vi "Revision Query.vi"(8 "error in (no error)":errorcluster, 11 "VISA resource name":refnum<visa-resource-name>) -> (0 "error out":errorcluster, 1 "Instrument Firmware Revision":string, 2 "Instrument Driver Revision":string, 3 "VISA resource name out":refnum<visa-resource-name>)   [LabVIEW 2018, in "Keithley 3706.lvlib"]
uses:
  <instrlib>/Keithley 3706/Keithley 3706.lvlib
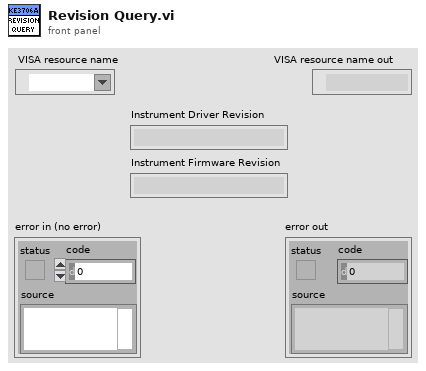
[diagram p1: front panel]
types:
  T1 = enum32{"invalid app kind", "Development System", "Run Time System", "Student Edition", "Embedded LabVIEW", "Evaluation", "Custom"}
  T2 = cluster{"Major":u16, "Minor":u16, "Fix":u16, "Build":u16}
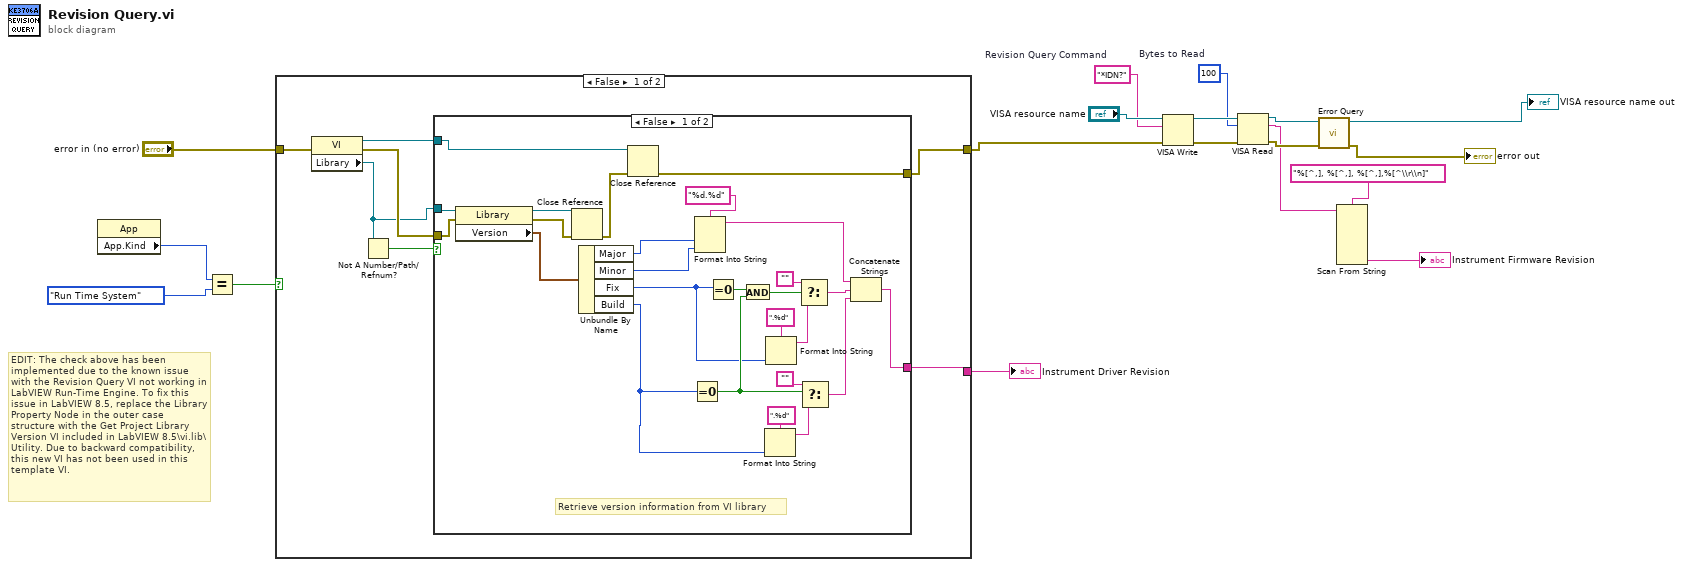
[diagram p0: block diagram]
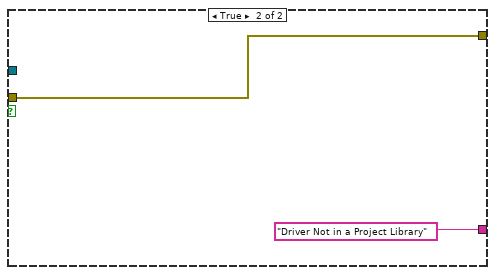
[diagram p2: hidden frame]
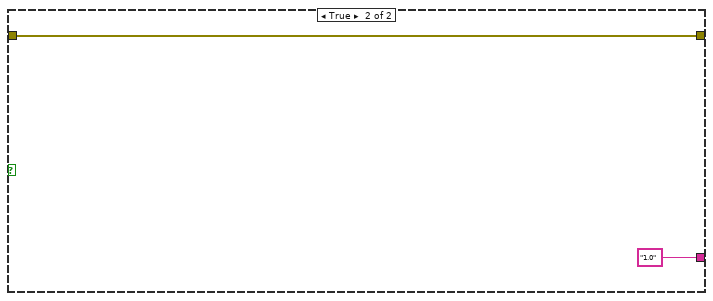
[diagram p3: hidden frame]
diagram:
  w8 = u32 100  # Bytes to Read
  w11 = "*IDN?"  # Revision Query Command
  # "EDIT: The check above has been implemented due to the known issue with the Revision Query VI not working in LabVIEW Run-Time Engine. To fix this issue in LabVIEW 8.5, replace the Library Property Node in the outer case structure with the Get Project Library Version VI included in LabVIEW 8.5\\vi.lib\\Utility. Due to backward compatibility, this new VI has not been used in this template VI."
  n1 = property class="App"() -> ("App.Kind"=w18:T1)  [unwired: 2 in, 2 out]
  n2 = Equal?(x=w18, y=T1."Run Time System" ("Application:Kind")) -> (x = y?=w16:bool)
  n3 = case shown="False" w16 {
    tunnel: "error in (no error)" -> [w25 w55]
    tunnel: [w20 w55] -> w13
    tunnel: [w21 "1.0"] -> w14
    frame False {
      n4 = property class="VI"(error in=w25) -> (reference out=w24:refnum<vi>, error out=w23:errorcluster, "Library"=w19:refnum<vi>)  [unwired: 1 in]
      n5 = Not A Number/Path/Refnum?(number/path/refnum=w19) -> (NaN/Path/Refnum?=w22:bool)
      n6 = case shown="False" w22 {
        tunnel: w24 -> [w47 _]
        tunnel: w23 -> [w51 w53]
        tunnel: [w45 w53] -> w20
        tunnel: [w39 "Driver Not in a Project Library"] -> w21
        tunnel: w19 -> [w50 _]
        frame False {
          # "Retrieve version information from VI library"
          n7 = property class="Library"(reference=w50, error in=w51) -> (reference out=w49:refnum<vi>, error out=w48:errorcluster, "Version"=w43:T2)
          n8 = Close Reference(reference=w49, error in (no error)=w48) -> (error out=w46:errorcluster)
          n9 = Unbundle By Name(w43) -> ("Major"=w42:u16, "Minor"=w41:u16, "Fix"=w28:u16, "Build"=w29:u16)
          n10 = Close Reference(reference=w47, error in (no error)=w46) -> (error out=w45:errorcluster)
          n11 = Equal To 0?(x=w29) -> (x = 0?=w37:bool)
          n12 = Format Into String(format string="%d.%d", w42, w41) -> (resulting string=w40:string)  [unwired: 2 in, 1 out]
          n13 = Equal To 0?(x=w28) -> (x = 0?=w36:bool)
          n14 = And(x=w36, y=w37) -> (x .and. y?=w38:bool)
          n15 = Format Into String(format string=".%d", w29) -> (resulting string=w33:string)  [unwired: 2 in, 1 out]
          n16 = Format Into String(format string=".%d", w28) -> (resulting string=w32:string)  [unwired: 2 in, 1 out]
          n17 = Select(t="", s=w38, f=w32) -> (s? t:f=w27:string)
          n18 = Select(t="", s=w37, f=w33) -> (s? t:f=w26:string)
          n19 = Concatenate Strings(w40, w27, w26) -> (w39:string)
        }
        frame True {
        }
      }
    }
    frame True {
    }
  }
  "Instrument Driver Revision" <- w14
  n20 = VISA Write(VISA resource name="VISA resource name", write buffer=w11, error in (no error)=w13) -> (VISA resource name out=w9:refnum<visa-resource-name>, error out=w10:errorcluster)  [unwired: 1 out]
  n21 = VISA Read(VISA resource name=w9, byte count=w8, error in (no error)=w10) -> (VISA resource name out=w7:refnum<visa-resource-name>, read buffer=w4:string, error out=w6:errorcluster)  [unwired: 1 out]
  n22 = call <instrlib>:"Error Query.vi"("error in (no error)"=w6, "VISA resource name"=w7) -> ("error out"=→"error out":errorcluster, "VISA resource name output"=→"VISA resource name out":refnum<visa-resource-name>)  [unwired: 6 in, 2 out]
  n23 = Scan From String(format string="%[^,], %[^,], %[^,],%[^\\r\\n]", input string=w4) -> (output 4=→"Instrument Firmware Revision":string)  [unwired: 9 in, 3 out]
